vi "DataLog Format Points File Path.vi"(0 "tag log directory":path, 7 "log file index":i32) -> (4 "dup tag log directory":path, 8 "log file path":path)   [LabVIEW 2012]
doc: "Format the name of the log file based on a log file index and tag log directory."
uses:
  glb_DataLog MCVD.vi
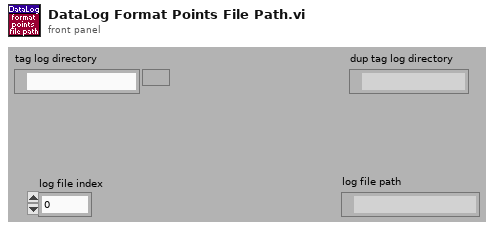
[diagram p1: front panel]
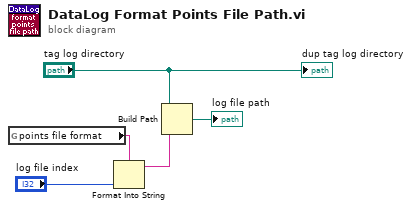
[diagram p0: block diagram]
diagram:
  n1 = global read "glb_DataLog MCVD.vi" "points file format"() -> (w4:string)
  n2 = Format Into String(format string=w4, "log file index") -> (resulting string=w3:string)  [unwired: 2 in, 1 out]
  n3 = Build Path(base path="tag log directory", name or relative path=w3) -> (appended path=→"log file path":path)
  "dup tag log directory" <- "tag log directory"
